vi "自動抓相機.vi"(8 "error in":errorcluster) -> (0 "error out":errorcluster, 3 "Session Out":T1)   [LabVIEW 2015]
uses:
  <vilib>/userdefined/High Color/IMAQdx.ctl
  <vilib>/vision/driver/NI_Vision_Acquisition_Software.lvlib
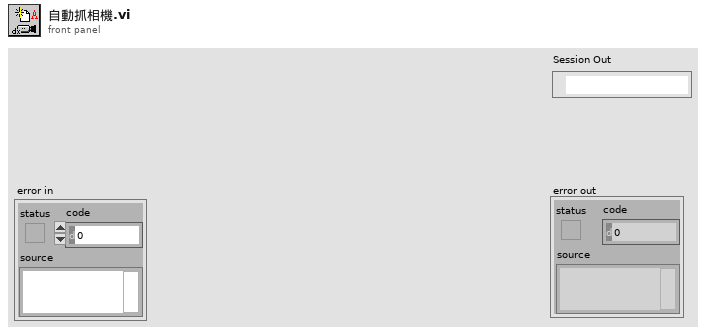
[diagram p1: front panel]
types:
  T1 = typedef "IMAQdx.ctl" = refnum<k21>
  T2 = cluster{"Type":u32, "Version":u32, "Flags":u32, "SerialNumberHigh":u32, "SerialNumberLow":u32, "BusType":u32, "InterfaceName":string, "VendorName":string, "ModelName":string, "CameraFileName":string, "CameraAttributeURL":string}[]
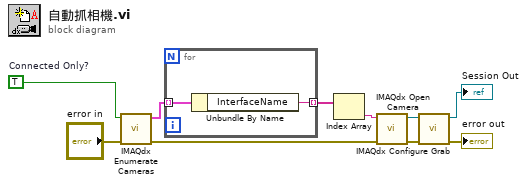
[diagram p0: block diagram]
diagram:
  w9 = TRUE  # Connected Only?
  n1 = call <vilib>:"IMAQdx Enumerate Cameras.vi"("error in"="error in", "Connected Only? (Yes)"=w9) -> ("error out"=w3:errorcluster, "Camera Information Array"=w10:T2)  [unwired: 8 out]
  n2 = for {
    tunnel: w10 -> [w12] mode=indexing
    tunnel: [w11] -> w8 mode=indexing
    n3 = Unbundle By Name(w12) -> ("InterfaceName"=w11:string)
  }
  n4 = Index Array(array=w8) -> (element=w4:string)  [unwired: 1 in]
  n5 = call <vilib>:"IMAQdx Open Camera.vi"("error in"=w3, "Session In"=w4) -> ("error out"=w6:errorcluster, "Session Out"=w5:T1)  [unwired: 1 in, 7 out]
  n6 = call <vilib>:"IMAQdx Configure Grab.vi"("error in"=w6, "Session In"=w5) -> ("error out"=→"error out":errorcluster, "Session Out"=→"Session Out":T1)  [unwired: 8 out]
